vi "Do.vi"(8 "error in (no error)":errorcluster, 10 "Actor in":refnum<class "Actor.lvclass">, 11 "Add Value without TS Msg":refnum<class "Add Value without TS Msg.lvclass">) -> (0 "error out":errorcluster, 2 "Actor out":refnum<class "Actor.lvclass">)   [LabVIEW 2019, in "BNT_XtGraph.lvlib" / "Add Value without TS Msg.lvclass"]
doc: "This VI delivers the message to the actor by calling the appropriate method(s) on the actor."
uses:
  Add Value without TS Msg.lvclass
  BNT_XtGraph/BNT_XtGraph.lvclass
  CSPP_Core/Messages/CSPP_PVUpdate Msg/CSPP_PVUpdate Msg.lvclass
  CSPP_Core/Classes/CSPP_ProcessVariables/ProcessVariable/PV.lvclass
  C:/Users/Holger/Documents/LVP/HEITRONICS/TempCtrl/Packages/CSPP_Core/Messages/CSPP_PVUpdate Msg/CSPP_PVUpdate Msg.lvclass
  C:/Users/Holger/Documents/LVP/HEITRONICS/TempCtrl/Packages/CSPP_Core/Messages/CSPP_AsyncCallbackMsg/CSPP_AsyncCallback Msg.lvclass
  C:/Program Files (x86)/National Instruments/LabVIEW 2018/vi.lib/ActorFramework/Message/Message.lvclass
  C:/Users/Holger/Documents/LVP/HEITRONICS/TempCtrl/Packages/CSPP_Core/Actors/CSPP_BaseActor/CSPP_BaseActor.lvclass
  C:/Program Files (x86)/National Instruments/LabVIEW 2018/vi.lib/ActorFramework/Actor/Actor.lvclass
  <vilib>/ActorFramework/Actor/Actor.lvclass
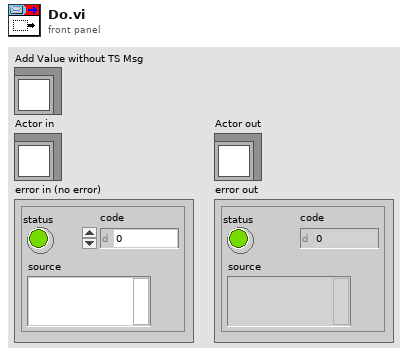
[diagram p1: front panel]
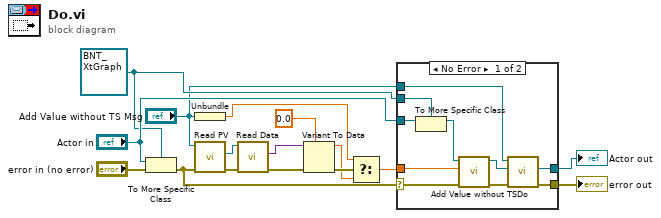
[diagram p0: block diagram]
diagram:
  w12 = refnum<class "BNT_XtGraph.lvclass"> refnum ("Actor in")
  n1 = To More Specific Class(target class=w12, reference="Actor in", error in="error in (no error)") -> (error out=w11:errorcluster)  [unwired: 1 out]
  n2 = Unbundle ("Pre-Unbundler")("Add Value without TS Msg") -> (w1:dbl)
  n3 = call "Read PV.vi"("error in (no error)"=w11, "CS++PVUpdate Msg in"="Add Value without TS Msg") -> ("error out"=w10:errorcluster, "PV"=w7:refnum<class "PV.lvclass">)  [unwired: 7 in, 1 out]
  n4 = call "Read Data.vi"("error in (no error)"=w10, "PV in"=w7) -> ("error out"=w4:errorcluster, "Data"=w3:variant)  [unwired: 7 in, 1 out]
  n5 = Variant To Data(error in=w4, type=0.0 ("Value"), Variant=w3) -> (data=w5:dbl, error out=w9:errorcluster)
  n6 = Select ("MainSelect")(t=w1, s=w9, f=w5) -> (s? t:f=w2:dbl)
  n7 = case shown="No Error" w11 {
    selector: w11 -> [w26 w28]
    tunnel: [w20 w28] -> w15
    tunnel: [w22 w27] -> w14
    tunnel: "Actor in" -> [w25 w27]
    tunnel: w12 -> [w24 _]
    tunnel: "Add Value without TS Msg" -> [w18 _]
    tunnel: w2 -> [w17 _]
    frame No Error {
      n8 = To More Specific Class ("To More Specific Class (internal)")(target class=w24, reference=w25) -> (specific class reference=w23:refnum<class "BNT_XtGraph.lvclass">)  [unwired: 1 in, 1 out]
      n9 = call "Add Value without TS.vi"("Error In"=w26, "Value"=w17, "BNT_XtGraph in"=w23) -> ("Error Out"=w19:errorcluster, "BNT_XtGraph out"=w21:refnum<class "BNT_XtGraph.lvclass">)  [unwired: 7 in]
      n10 = call-parent "Do.vi"("error in (no error)"=w19, "Actor in"=w21, "CS++PVUpdate Msg"=w18) -> ("error out"=w20:errorcluster, "Actor out"=w22:refnum<class "Actor.lvclass">)  [unwired: 7 in]
    }
    frame Error {
    }
  }
  "error out" <- w15
  "Actor out" <- w14
